vi "Add VI from Ref.vi"(8 "error in (no error)":errorcluster, 10 "VI Ref":refnum<vi>, 11 "Model in":refnum<class "Model.lvclass">) -> (0 "error out":errorcluster, 3 "Model out":refnum<class "Model.lvclass">)   [LabVIEW 2015, in "Model.lvlib" / "Model.lvclass"]
uses:
  Model.lvclass
  Controls/VI Infomation.ctl
  Model.lvlib
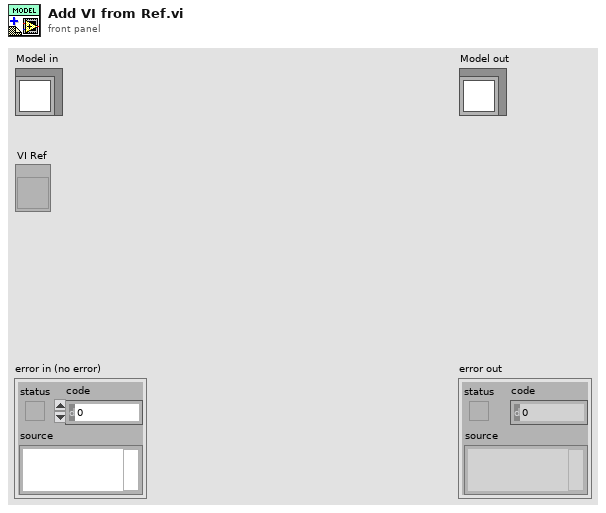
[diagram p1: front panel]
types:
  T1 = typedef "Model.lvlib/VI Infomation.ctl" = cluster{"Name":string, "Description":string, "Icon":picture}
  T2 = typedef "imagedata.ctl" = cluster{"image type":i32, "image depth":i32, "image":u8[], "mask":u8[], "colors":u32[], "Rectangle":cluster{"left":i16, "top":i16, "right":i16, "bottom":i16}}
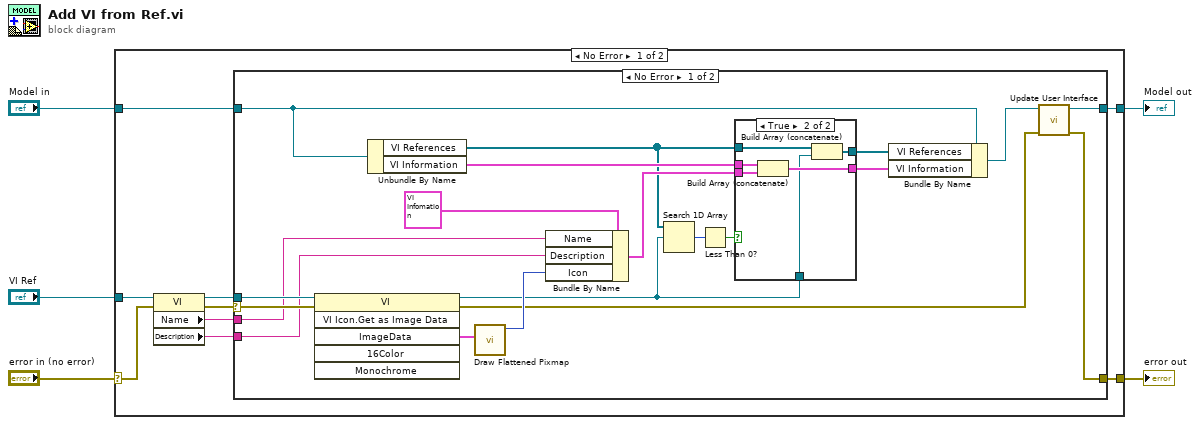
[diagram p0: block diagram]
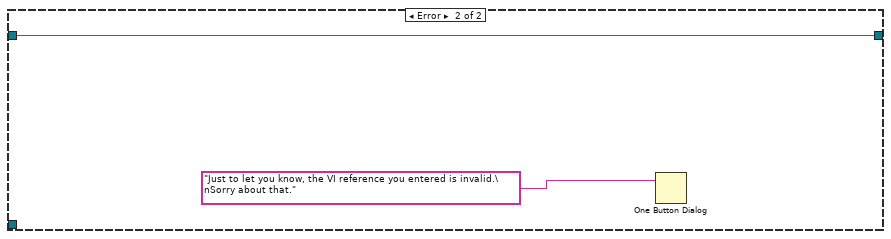
[diagram p3: hidden frame]
diagram:
  n1 = case shown="No Error" "error in (no error)" {
    selector: "error in (no error)" -> [w10 w46]
    tunnel: [w6 w46] -> w4
    tunnel: [w7 w45] -> w2
    tunnel: "Model in" -> [w9 w45]
    tunnel: "VI Ref" -> [w8 _]
    frame No Error {
      n2 = property class="VI"(reference=w8, error in=w10) -> (reference out=w14:refnum<vi>, error out=w13:errorcluster, "Name"=w12:string, "Description"=w11:string)
      n3 = case shown="No Error" w13 {
        selector: w13 -> [w32 _]
        tunnel: w14 -> [w33 _]
        tunnel: w12 -> [w31 _]
        tunnel: w11 -> [w30 _]
        tunnel: w9 -> [w23 w44]
        tunnel: [w21 w44] -> w7
        tunnel: [w19 _] -> w6
        frame No Error {
          n4 = invoke class="VI" method="VI Icon.Get as Image Data"(reference=w33, error in=w32) -> (reference out=w17:refnum<vi>, error out=w20:errorcluster, "ImageData"=w34:T2)  [unwired: 4 in, 3 out]
          n5 = Unbundle By Name(w23) -> ("VI References"=w18:refnum<vi>[], "VI Information"=w26:T1[])
          n6 = call <vilib>:"Draw Flattened Pixmap.vi"("image data"=w34) -> ("new picture"=w29:picture)  [unwired: 8 in]
          n7 = Bundle By Name(cluster=T1 {"Name"="", "Description"="", "Icon"=bytes[0]} ("VI Infomation"), "Name"=w31, "Description"=w30, "Icon"=w29) -> (w27:T1)
          n8 = Search 1D Array(1D array=w18, element=w17) -> (index of element=w16:i32)  [unwired: 1 in]
          n9 = Less Than 0?(x=w16) -> (x < 0?=w15:bool)
          n10 = case shown="True" w15 {
            tunnel: w27 -> [_ w42]
            tunnel: w26 -> [w35 w41]
            tunnel: [w36 w40] -> w25
            tunnel: [w35 w39] -> w24
            tunnel: w18 -> [w36 w38]
            tunnel: w17 -> [_ w37]
            frame False {
            }
            frame True {
              n11 = Build Array (concatenate)(w41, w42) -> (w39:T1[])
              n12 = Build Array (concatenate)(w38, w37) -> (w40:refnum<vi>[])
            }
          }
          n13 = Bundle By Name(cluster=w23, "VI References"=w25, "VI Information"=w24) -> (w22:refnum<class "Model.lvclass">)
          n14 = call "Update User Interface.vi"("error in (no error)"=w20, "Model in"=w22) -> ("error out"=w19:errorcluster, "Model out"=w21:refnum<class "Model.lvclass">)  [unwired: 8 in]
        }
        frame Error {
          n15 = One Button Dialog(message="Just to let you know, the VI reference you entered is invalid.\nSorry about that.") -> ()  [unwired: 1 in, 1 out]
        }
      }
    }
    frame Error {
    }
  }
  "error out" <- w4
  "Model out" <- w2
